vi "Combine Status Monitor and Transient Capture.vi"() -> ()   [LabVIEW 2017]
uses:
  Status Monitor/Status Monitor (Single Unit).vi
  Status Monitor/Status Monitor Library.lvlib
panel:
  out "UUT Name":string
  in  "Soft Trigger":bool
  in  "Post-Trigger Samples":i32=100000
  in  "configuration file path":path
  in  "stop":bool
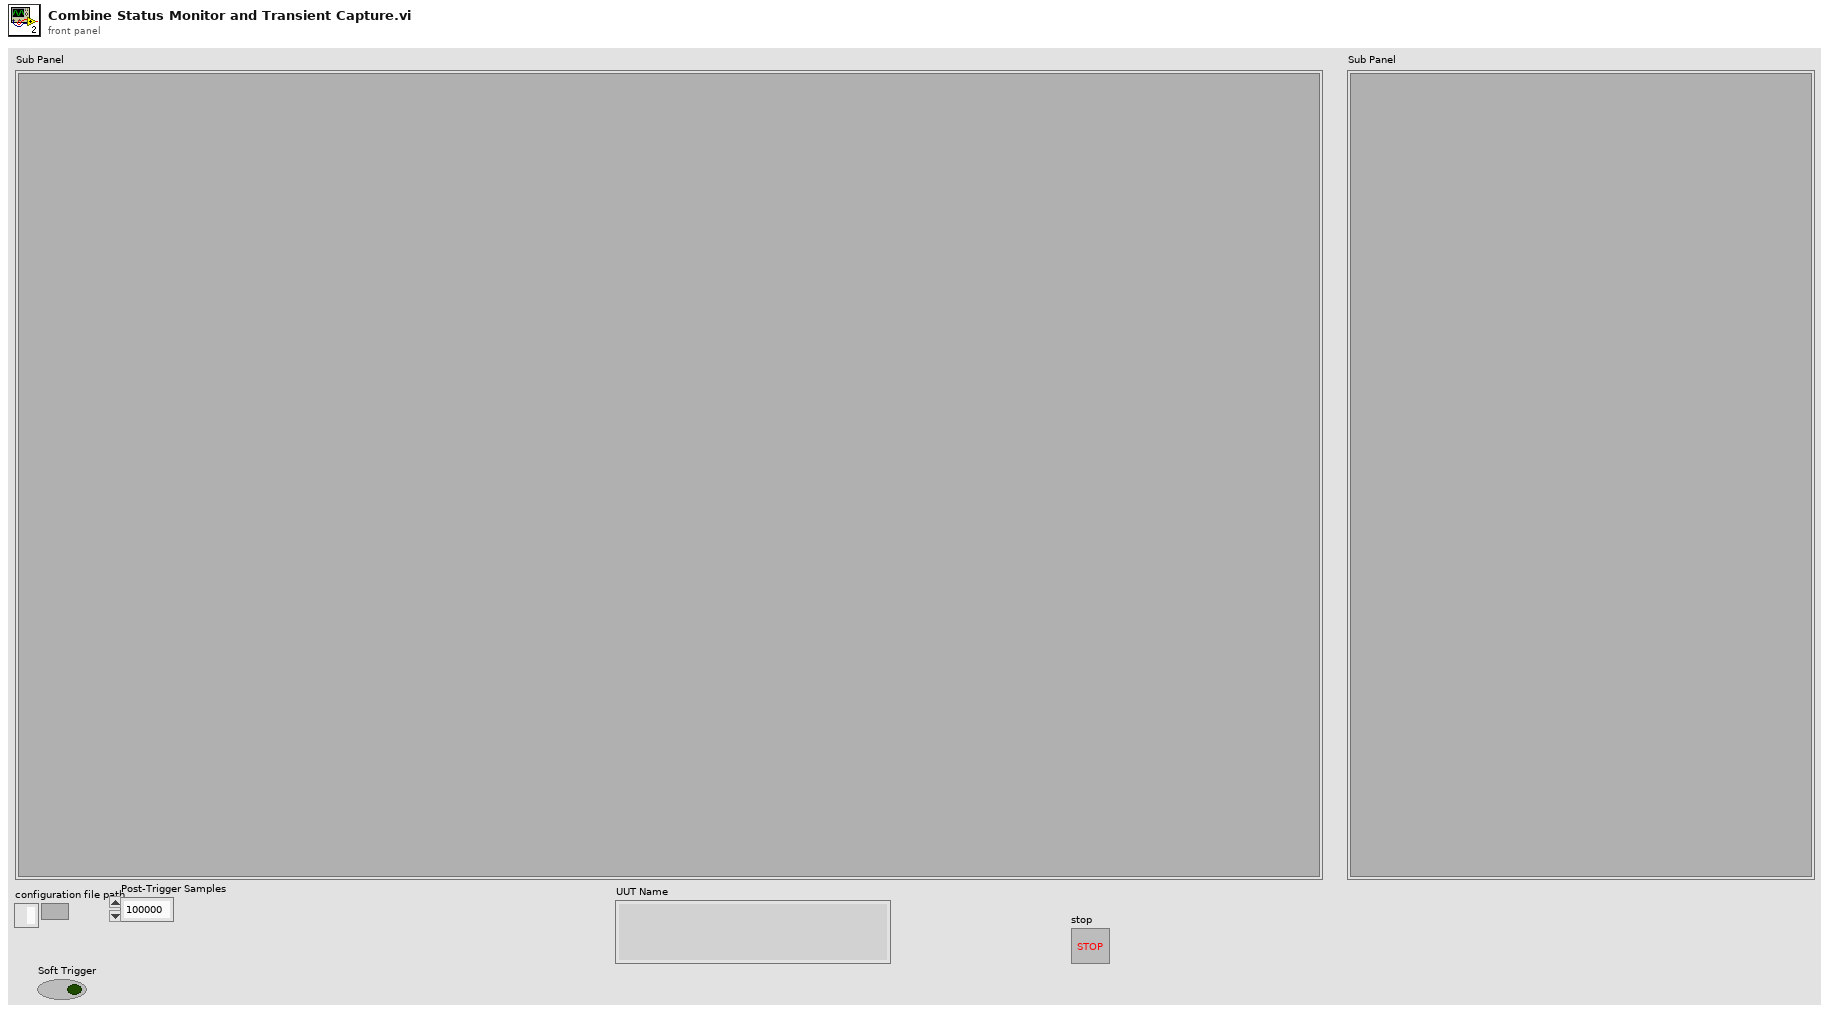
[diagram p1: front panel]
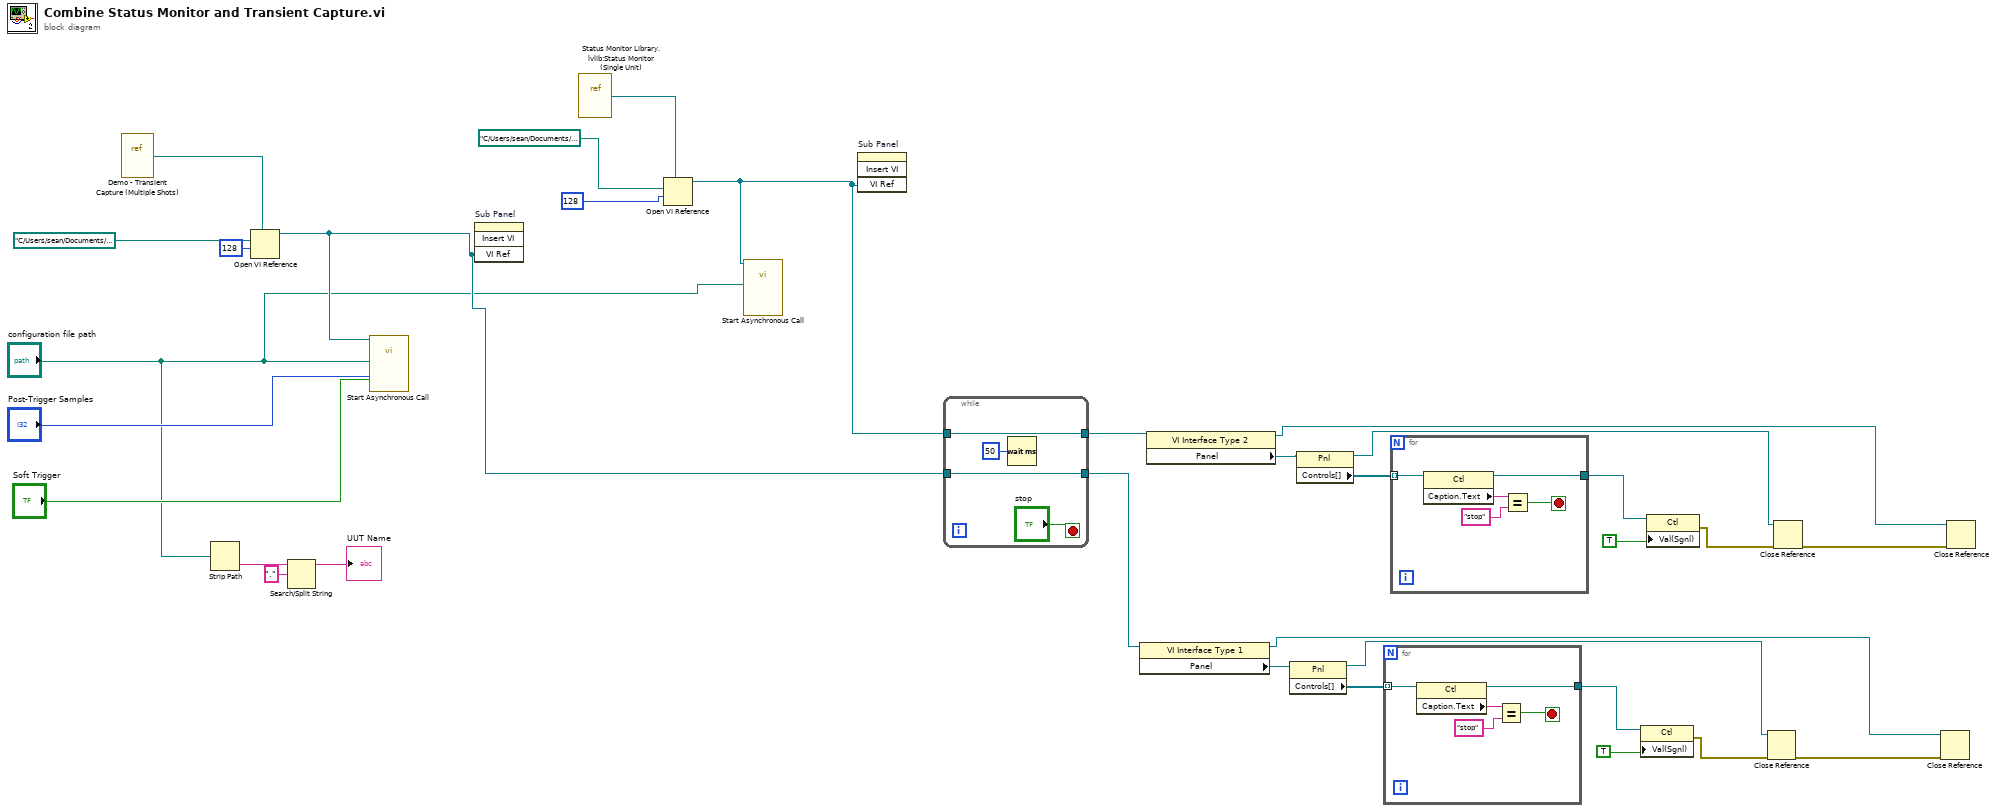
[diagram p0: block diagram]
diagram:
  n1 = vi-ref "Demo - Transient Capture (Multiple Shots).vi"() -> (w30:refnum<vi>)
  n2 = Strip Path(path="configuration file path") -> (name=w20:string)  [unwired: 1 out]
  n3 = Open VI Reference(type specifier VI Refnum (for type only)=w30, vi path=path "C:/Users/sean/Documents/Workspace/LabVIEW/Sean/acq400_lv/Source Code/Transient Capture (Advanced Demo)/Demo - Transient Capture (Multiple Shots).vi", options=128) -> (vi reference=w31:refnum<vi>)  [unwired: 3 in, 1 out]
  n4 = Search/Split String(string=w20, search string/char (-)=".") -> (substring before match=→"UUT Name":string)  [unwired: 1 in, 2 out]
  n5 = call-by-ref "Start Asynchronous Call"(reference=w31, "Soft Trigger"="Soft Trigger", "Post-Trigger Samples"="Post-Trigger Samples", "configuration file path"="configuration file path") -> ()  [unwired: 10 in, 2 out]
  n6 = invoke on="Sub Panel" class="SubPnl" method="Insert VI"("VI Ref"=w31) -> ()  [unwired: 3 in, 4 out]
  n7 = vi-ref "Status Monitor Library.lvlib:Status Monitor (Single Unit).vi"() -> (w27:refnum<vi>)
  n8 = Open VI Reference(type specifier VI Refnum (for type only)=w27, vi path=path "C:/Users/sean/Documents/Workspace/LabVIEW/Sean/acq400_lv/Source Code/Status Monitor/Status Monitor (Single Unit).vi", options=128) -> (vi reference=w26:refnum<vi>)  [unwired: 3 in, 1 out]
  n9 = call-by-ref "Start Asynchronous Call"(reference=w26, "configuration file path"="configuration file path") -> ()  [unwired: 12 in, 2 out]
  n10 = invoke on="Sub Panel" class="SubPnl" method="Insert VI"("VI Ref"=w26) -> ()  [unwired: 3 in, 4 out]
  n11 = while {
    tunnel: w26 -> [w36]
    tunnel: w31 -> [w35]
    tunnel: [w36] -> w18
    tunnel: [w35] -> w3
    stop <- "stop" stop-if-true
    n12 = Wait (ms)(milliseconds to wait=u32 50) -> ()  [unwired: 1 out]
  }
  n13 = property class="VI Interface Type 1"(reference=w3) -> (reference out=w5:refnum<vi>, "Panel"=w9:refnum<vi>)  [unwired: 1 in, 1 out]
  n14 = property class="VI Interface Type 2"(reference=w18) -> (reference out=w11:refnum<vi>, "Panel"=w17:refnum<vi>)  [unwired: 1 in, 1 out]
  n15 = property class="Pnl"(reference=w9) -> (reference out=w6:refnum<vi>, "Controls[]"=w2:refnum<vi>[])  [unwired: 1 in, 1 out]
  n16 = property class="Pnl"(reference=w17) -> (reference out=w12:refnum<vi>, "Controls[]"=w16:refnum<vi>[])  [unwired: 1 in, 1 out]
  n17 = for {
    tunnel: w2 -> [w41] mode=indexing
    tunnel: [w37] -> w8
    stop <- w38 stop-if-true
    n18 = property class="Ctl"(reference=w41) -> (reference out=w37:refnum<vi>, "Caption.Text"=w40:string)  [unwired: 1 in, 1 out]
    n19 = Equal?(x=w40, y="stop") -> (x = y?=w38:bool)
  }
  n20 = for {
    tunnel: w16 -> [w46] mode=indexing
    tunnel: [w42] -> w15
    stop <- w43 stop-if-true
    n21 = property class="Ctl"(reference=w46) -> (reference out=w42:refnum<vi>, "Caption.Text"=w45:string)  [unwired: 1 in, 1 out]
    n22 = Equal?(x=w45, y="stop") -> (x = y?=w43:bool)
  }
  n23 = property class="Ctl"(reference=w8, "Val(Sgnl)"=TRUE) -> (error out=w1:errorcluster)  [unwired: 1 in, 1 out]
  n24 = property class="Ctl"(reference=w15, "Val(Sgnl)"=TRUE) -> (error out=w13:errorcluster)  [unwired: 1 in, 1 out]
  n25 = Close Reference(reference=w6, error in (no error)=w1) -> (error out=w4:errorcluster)
  n26 = Close Reference(reference=w12, error in (no error)=w13) -> (error out=w10:errorcluster)
  n27 = Close Reference(reference=w5, error in (no error)=w4) -> ()  [unwired: 1 out]
  n28 = Close Reference(reference=w11, error in (no error)=w10) -> ()  [unwired: 1 out]
